vi "contar.vi"(8 "error in (no error)":errorcluster, 9 "Max":u8, 10 "Cuenta":u8, 11 "ContadorB in":refnum<class "ContadorB.lvclass">) -> (0 "error out":errorcluster, 3 "ContadorB out":refnum<class "ContadorB.lvclass">)   [LabVIEW 2019, in "ContadorB.lvlib" / "ContadorB.lvclass"]
uses:
  ContadorB.lvclass
  ContadorB.lvclass/ContadorB.ctl
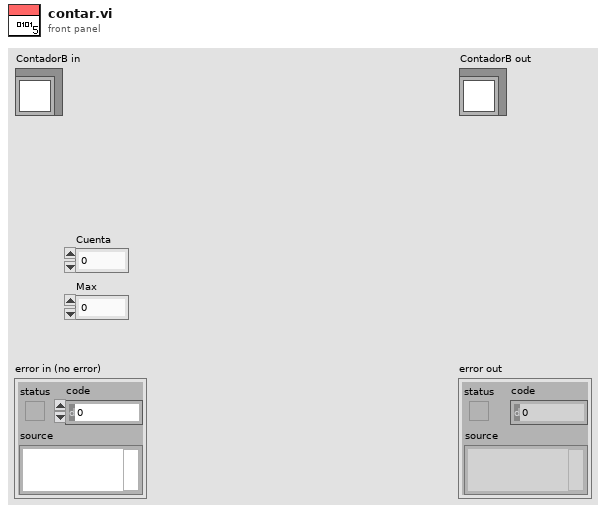
[diagram p1: front panel]
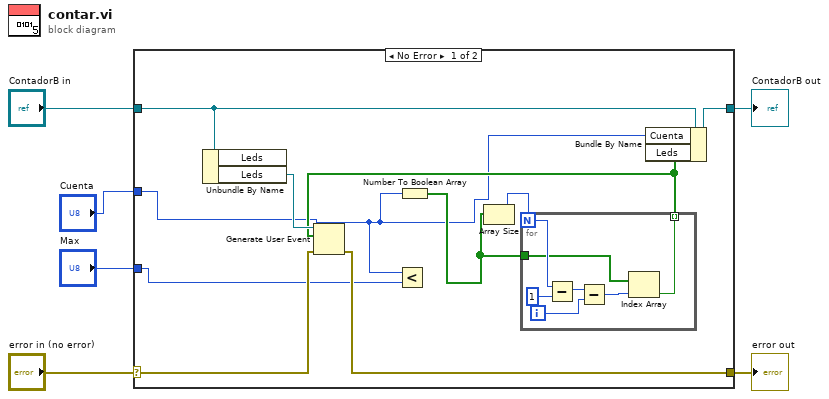
[diagram p0: block diagram]
diagram:
  n1 = case shown="No Error" "error in (no error)" {
    selector: "error in (no error)" -> [w12 w25]
    tunnel: [w11 w25] -> w5
    tunnel: [w15 w24] -> w3
    tunnel: "ContadorB in" -> [w16 w24]
    tunnel: "Cuenta" -> [w8 _]
    tunnel: "Max" -> [w9 _]
    frame No Error {
      n2 = Unbundle By Name(w16) -> ("Leds"=w13:refnum<user-event>)  [unwired: 1 out]
      n3 = Less?(x=w8, y=w9) -> ()  [unwired: 1 out]
      n4 = Number To Boolean Array(number=w8) -> (Boolean array=w14:bool[])
      n5 = Array Size(array=w14) -> (size(s)=w7:i32)
      n6 = for {
        N: w7 -> [w23]
        tunnel: w14 -> [w18]
        tunnel: [w17] -> w10 mode=indexing
        i -> [w20]
        n7 = Subtract(x=w23, y=1) -> (x-y=w21:i32)
        n8 = Subtract(x=w21, y=w20) -> (x-y=w19:i32)
        n9 = Index Array(array=w18, index=w19) -> (element=w17:bool)
      }
      n10 = Generate User Event(user event=w13, event data cluster=w10, error in=w12) -> (error out=w11:errorcluster)  [unwired: 1 in, 1 out]
      n11 = Bundle By Name(cluster=w16, "Cuenta"=w8, "Leds"=w10) -> (w15:refnum<class "ContadorB.lvclass">)
    }
    frame Error {
    }
  }
  "error out" <- w5
  "ContadorB out" <- w3
